vi "BuildMenu.vi"(0 "XRef":T7, 1 "MenuRef":T6, 2 "Point":T4, 3 "Menu Type":T3, 4 "State In":T2) -> (14 "Fatal Error Out":T1)   [LabVIEW 2015, in "LVJSON.lvlib" / "Index JSON Array.xnode"]
uses:
  Index JSON Array.xnode
  <vilib>/XNodeSupport/XNodeXNodeRef.ctl
  <vilib>/XNodeSupport/XNodeMenuRef.ctl
  <vilib>/XNodeSupport/XNodePoint.ctl
  <vilib>/XNodeSupport/XNodeInt.ctl
  <vilib>/XNodeSupport/XNodeMenuType.ctl
  State.ctl
  <vilib>/XNodeSupport/XNodeErrorCluster.ctl
  dimensions.vi
  <vilib>/XNodeSupport/NI_XNodeSupport.lvlib
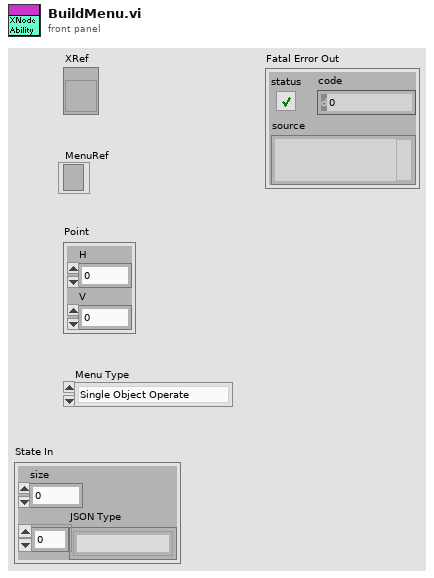
[diagram p1: front panel]
types:
  T1 = typedef "NI_XNodeSupport.lvlib/XNodeErrorCluster.ctl" = errorcluster
  T2 = typedef "LVJSON.lvlib/Index JSON Array.xnode/State.ctl" = cluster{"size":u32, "JSON Type":string[]}
  T3 = typedef "NI_XNodeSupport.lvlib/XNodeMenuType.ctl" = enum32{"Single Object Operate", "Single Object Popup", "Multi Object Popup Master", "Multi Object Popup Other"}
  T4 = typedef "NI_XNodeSupport.lvlib/XNodePoint.ctl" = cluster{"H":T5, "V":T5}
  T5 = typedef "NI_XNodeSupport.lvlib/XNodeInt.ctl" = i32
  T6 = typedef "NI_XNodeSupport.lvlib/XNodeMenuRef.ctl" = refnum<k9>
  T7 = typedef "NI_XNodeSupport.lvlib/XNodeXNodeRef.ctl" = refnum<vi>
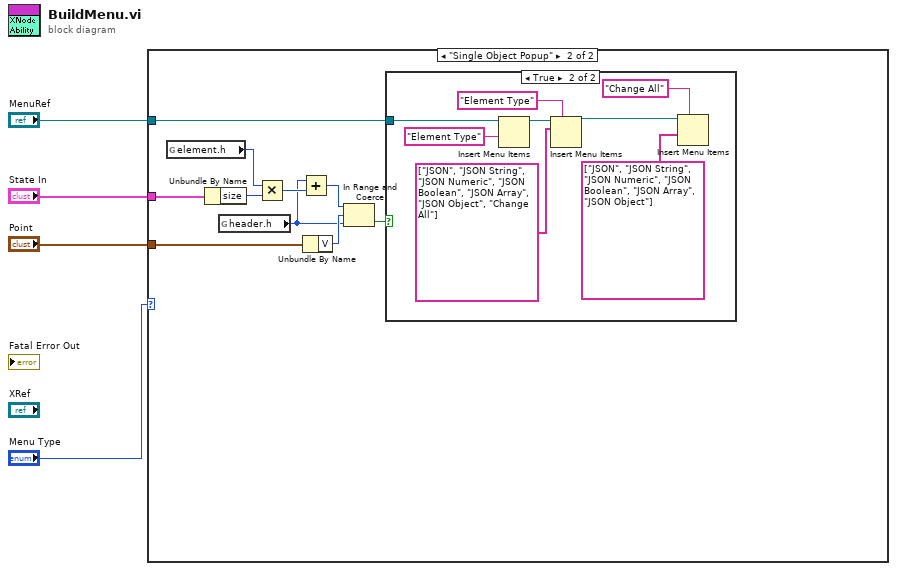
[diagram p0: block diagram]
diagram:
  n1 = case shown="\"Single Object Popup\"" "Menu Type" {
    tunnel: "MenuRef" -> [_ w14]
    tunnel: "Point" -> [_ w13]
    tunnel: "State In" -> [_ w12]
    frame "Single Object Operate", Default {
    }
    frame "Single Object Popup" {
      n2 = global read "dimensions.vi" "element.h"() -> (w10:i16)
      n3 = Unbundle By Name(w12) -> ("size"=w11:u32)
      n4 = global read "dimensions.vi" "header.h"() -> (w5:i16)
      n5 = Multiply(x=w10, y=w11) -> (x*y=w9:u32)
      n6 = Add(x=w5, y=w9) -> (x+y=w6:u32)
      n7 = Unbundle By Name(w13) -> ("V"=w7:T5)
      n8 = In Range and Coerce(upper limit=w6, x=w7, lower limit=w5) -> (In Range?=w8:bool)  [unwired: 1 out]
      n9 = case shown="True" w8 {
        tunnel: w14 -> [_ w20]
        frame False {
        }
        frame True {
          n10 = Insert Menu Items(7:"Element Type", 9:w20) -> (3:w18:refnum<k9>)  [unwired: 4 in, 2 out]
          n11 = Insert Menu Items(5:"Element Type" ("menu tag"), 8:string[] ["JSON", "JSON String", "JSON Numeric", "JSON Boolean", "JSON Array", "JSON Object", "Change All"] ("item names"), 9:w18) -> (3:w17:refnum<k9>)  [unwired: 3 in, 2 out]
          n12 = Insert Menu Items(5:"Change All" ("menu tag"), 7:string[] ["JSON", "JSON String", "JSON Numeric", "JSON Boolean", "JSON Array", "JSON Object"] ("item names"), 9:w17) -> ()  [unwired: 3 in, 3 out]
        }
      }
    }
  }
